vi "ProcessDeviationMeasurementResults.vi"(0 "Peak detected?":bool, 5 "Callibration Peak Position":dbl, 7 "Measurement Peak Position":dbl, 9 "Refractive index":dbl, 11 "Compensation factor":dbl, 12 "Wanted thickness":dbl, 13 "Thickness range":dbl) -> (4 "Lens thickness in range?":bool, 6 "Lens thickness":dbl)   [LabVIEW 2013]
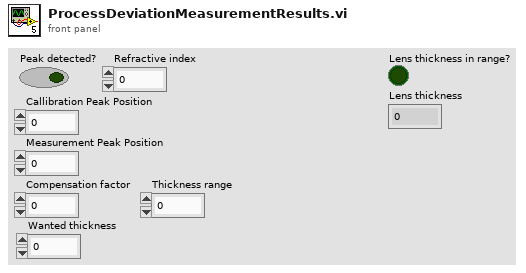
[diagram p1: front panel]
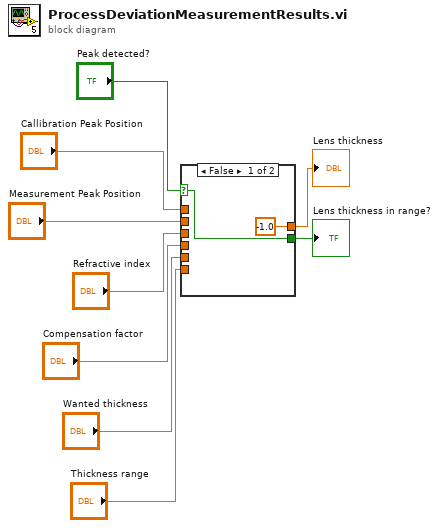
[diagram p0: block diagram]
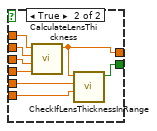
[diagram p2: hidden frame]
diagram:
  n1 = case shown="False" "Peak detected?" {
    selector: "Peak detected?" -> [w11 _]
    tunnel: [w11 w19] -> w8
    tunnel: [-1.0 ("Lens thickness") w18] -> w7
    tunnel: "Wanted thickness" -> [_ w17]
    tunnel: "Thickness range" -> [_ w16]
    tunnel: "Callibration Peak Position" -> [_ w15]
    tunnel: "Measurement Peak Position" -> [_ w14]
    tunnel: "Refractive index" -> [_ w13]
    tunnel: "Compensation factor" -> [_ w12]
    frame False {
    }
    frame True {
      n2 = call "CalculateLensThickness.vi"("Compensation factor"=w12, "Refractive index"=w13, "Measurement Peak Position"=w14, "Callibration Peak Position"=w15) -> ("Lens thickness"=w18:dbl)  [unwired: 7 in]
      n3 = call "CheckIfLensThicknessInRange.vi"("Thickness range"=w16, "Wanted thickness"=w17, "Lens thickness"=w18) -> ("Lens thickness in range?"=w19:bool)  [unwired: 8 in]
    }
  }
  "Lens thickness in range?" <- w8
  "Lens thickness" <- w7
